vi "Auto Settings.vi"(0 "Mid Switch Forward Time":dbl=1.0 min=0.0, 1 "Mid Switch Strafe Time":dbl=1.0 min=0.0, 2 "Mid Switch Forward Speed":dbl=1.0 min=-1.0 max=1.0, 3 "Mid Switch Strafe Speed":dbl=1.0 min=-1.0 max=1.0, 7 "Strafe From Wall Time":dbl=1.0 min=0.0, 10 "Strafe From Wall Speed":dbl=1.0 min=-1.0 max=1.0) -> ()   [LabVIEW 2017]
uses:
  <vilib>/Rock Robotics/Network Tables/NT Write Number.vi
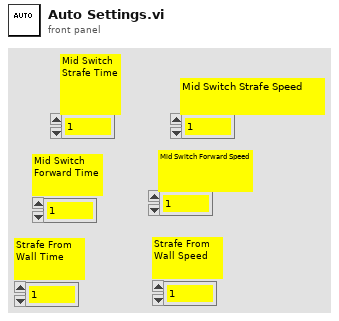
[diagram p1: front panel]
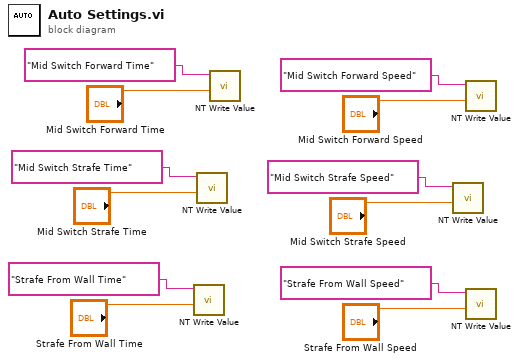
[diagram p0: block diagram]
diagram:
  n1 = call-poly <vilib>:"NT Write Value.vi"("Numeric"="Strafe From Wall Time", "Name"="Strafe From Wall Time") -> ()  [unwired: 9 in, 1 out]
  n2 = call-poly <vilib>:"NT Write Value.vi"("Numeric"="Mid Switch Strafe Time", "Name"="Mid Switch Strafe Time") -> ()  [unwired: 9 in, 1 out]
  n3 = call-poly <vilib>:"NT Write Value.vi"("Numeric"="Mid Switch Forward Time", "Name"="Mid Switch Forward Time") -> ()  [unwired: 9 in, 1 out]
  n4 = call-poly <vilib>:"NT Write Value.vi"("Numeric"="Mid Switch Strafe Speed", "Name"="Mid Switch Strafe Speed") -> ()  [unwired: 9 in, 1 out]
  n5 = call-poly <vilib>:"NT Write Value.vi"("Numeric"="Mid Switch Forward Speed", "Name"="Mid Switch Forward Speed") -> ()  [unwired: 9 in, 1 out]
  n6 = call-poly <vilib>:"NT Write Value.vi"("Numeric"="Strafe From Wall Speed", "Name"="Strafe From Wall Speed") -> ()  [unwired: 9 in, 1 out]
